vi "Print Console.vi"() -> ()   [LabVIEW 2018]
doc: "인쇄 작업 제출을 컨트롤하고 인쇄 작업의 처리 상태를 모니터"
uses:
  <vilib>/Utility/error.llb/DialogType.ctl
panel:
  out "인쇄 인디케이터":T1={"대기 중"=TRUE, "초기화 중"=FALSE, "인쇄 중"=FALSE, "작업 개수"=""}
  in  "정지 버튼":bool
  in  "큐 이벤트":bool
  out "큐 인쇄 작업":i32(slide) scale=0.0..25.0
  # "큐 인쇄 작업"
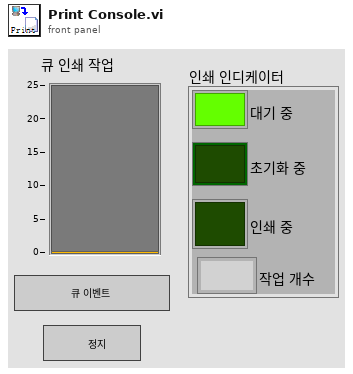
[diagram p1: front panel]
types:
  T1 = cluster{"대기 중":bool, "초기화 중":bool, "인쇄 중":bool, "작업 개수":string}
  T2 = typedef "DialogType.ctl" = u16
  T3 = enum16{"대기", "셋업 초기화", "셋업", "인쇄 초기화", "인쇄", "종료"}
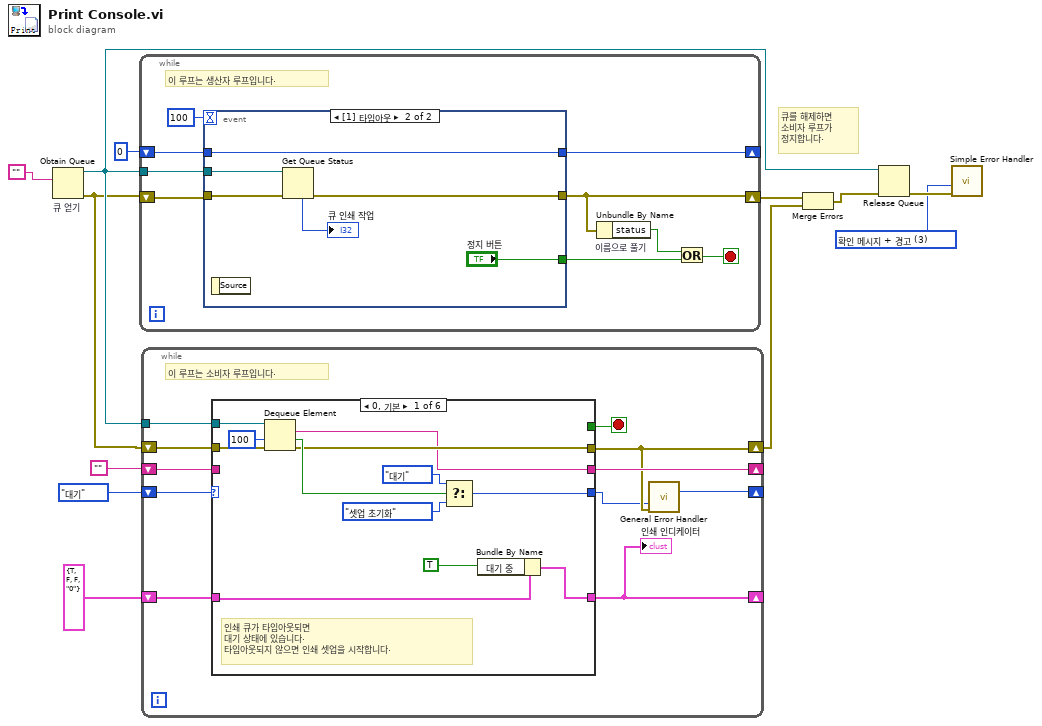
[diagram p0: block diagram]
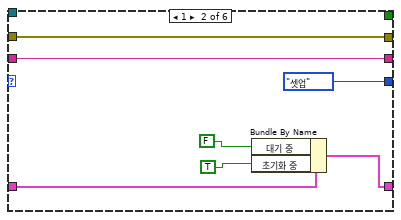
[diagram p2: hidden frame]
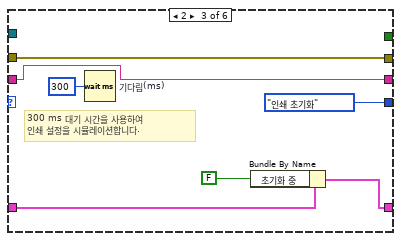
[diagram p3: hidden frame]
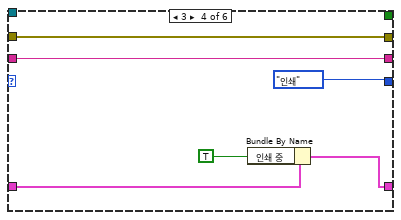
[diagram p4: hidden frame]
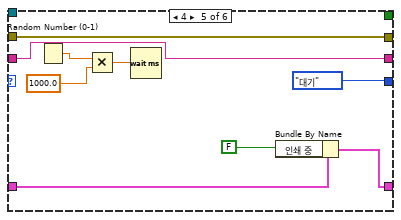
[diagram p5: hidden frame]
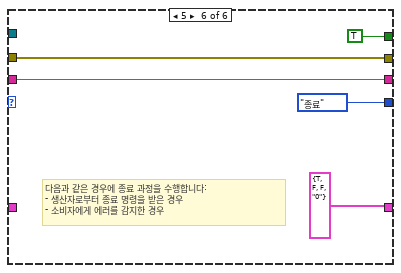
[diagram p6: hidden frame]
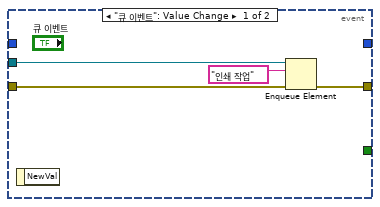
[diagram p7: hidden frame]
diagram:
  w1 = T2 3 items=["대화 상자 없음", "확인 메시지", "메시지 지속 또는 정지", "확인 메시지 + 경고", "지속/정지 + 경고"] ("type of dialog (OK msg:1)")
  # "큐를 해제하면\n소비자 루프가\n정지합니다."
  n1 = Obtain Queue "큐 얻기"(element data type="") -> (queue out=w11:refnum<queue>, error out=w6:errorcluster)  [unwired: 4 in, 1 out]
  n2 = while {
    tunnel: w11 -> [w20]
    shift-right: [w17] -> w5
    shift-left: w6 -> [w19]
    shift-right: [w13] -> _
    shift-left: 0 -> [w14]
    stop <- w18 stop-if-true
    # "이 루프는 생산자 루프입니다."
    n3 = event shown="[1] 타임아웃" {
      selector: _ -> [_ _]
      dyn-events: _ -> [_ _]
      timeout: 100 -> [_ _]
      tunnel: w20 -> [w24 w31]
      tunnel: w19 -> [w23 w30]
      tunnel: [w22 w29] -> w17
      tunnel: [_ "정지 버튼"] -> w15
      tunnel: [_ w27] -> w13
      tunnel: w14 -> [_ w27]
      event "큐 이벤트": Value Change {
        n4 = event-data() -> ()  [unwired: 1 in, 1 out]
        n5 = Enqueue Element(queue=w24, element="인쇄 작업" ("원소"), error in (no error)=w23) -> (error out=w22:errorcluster)  [unwired: 1 in, 2 out]
      }
      event Timeout {
        n6 = event-data() -> ()  [unwired: 1 in, 1 out]
        n7 = Get Queue Status(queue=w31, error in (no error)=w30) -> (error out=w29:errorcluster, # elements in queue=→"큐 인쇄 작업":i32)  [unwired: 1 in, 6 out]
      }
    }
    n8 = Unbundle By Name "이름으로 풀기"(w17) -> ("status"=w16:bool)
    n9 = Or(x=w16, y=w15) -> (x .or. y?=w18:bool)
  }
  n10 = while {
    shift-right: [w39] -> _
    shift-left: T1 {"대기 중"=TRUE, "초기화 중"=FALSE, "인쇄 중"=FALSE, "작업 개수"="0"} ("에러 상수") -> [w40]
    shift-right: [w32] -> _
    shift-left: T3."대기" -> [w42]
    tunnel: w11 -> [w41]
    shift-right: [w37] -> _
    shift-left: "" -> [w36]
    shift-right: [w34] -> w3
    shift-left: w6 -> [w38]
    stop <- w35 stop-if-true
    # "이 루프는 소비자 루프입니다."
    n11 = case shown="0, 기본" w42 {
      tunnel: w41 -> [w53 _ _ _ _ _]
      tunnel: [w52 enum16{"대기", "셋업 초기화", "셋업", "인쇄 초기화", "인쇄"}."셋업" enum16{"대기", "셋업 초기화", "셋업", "인쇄 초기화", "인쇄"}."인쇄 초기화" enum16{"대기", "셋업 초기화", "셋업", "인쇄 초기화", "인쇄"}."인쇄" enum16{"대기", "셋업 초기화", "셋업", "인쇄 초기화", "인쇄"}."대기" T3."종료"] -> w33
      tunnel: [w48 w57 w65 w72 w79 T1 {"대기 중"=TRUE, "초기화 중"=FALSE, "인쇄 중"=FALSE, "작업 개수"="0"} ("에러 상수")] -> w39
      tunnel: w40 -> [w47 w60 w66 w73 w80 _]
      tunnel: w38 -> [w45 w56 w63 w70 w76 w86]
      tunnel: [w44 w56 w63 w70 w76 w86] -> w34
      tunnel: [w43 w55 w62 w69 w75 w87] -> w37
      tunnel: w36 -> [_ w55 w62 w69 w75 w87]
      tunnel: [_ _ _ _ _ TRUE] -> w35
      frame 0, Default {
        # "인쇄 큐가 타임아웃되면\n대기 상태에 있습니다.\n타임아웃되지 않으면 인쇄 셋업을 시작합니다."
        n12 = Dequeue Element(queue=w53, timeout in ms (-1)=100 ("타임아웃(ms) (-1)"), error in (no error)=w45) -> (element=w43:string, timed out?=w51:bool, error out=w44:errorcluster)  [unwired: 1 out]
        n13 = Select(t=enum16{"대기", "셋업 초기화", "셋업", "인쇄 초기화", "인쇄"}."대기", s=w51, f=enum16{"대기", "셋업 초기화", "셋업", "인쇄 초기화", "인쇄"}."셋업 초기화") -> (s? t:f=w52:enum16{"대기", "셋업 초기화", "셋업", "인쇄 초기화", "인쇄"})
        n14 = Bundle By Name(cluster=w47, "대기 중"=TRUE) -> (w48:T1)
      }
      frame 1 {
        n15 = Bundle By Name(cluster=w60, "대기 중"=FALSE, "초기화 중"=TRUE) -> (w57:T1)
      }
      frame 2 {
        # "300 ms 대기 시간을 사용하여\n인쇄 설정을 시뮬레이션합니다."
        n16 = Wait (ms) "기다림(ms)"(milliseconds to wait=u32 300 ("대기 시간 (ms)")) -> ()  [unwired: 1 out]
        n17 = Bundle By Name(cluster=w66, "초기화 중"=FALSE) -> (w65:T1)
      }
      frame 3 {
        n18 = Bundle By Name(cluster=w73, "인쇄 중"=TRUE) -> (w72:T1)
      }
      frame 4 {
        n19 = Random Number (0-1)() -> (number: 0 to 1=w83:dbl)
        n20 = Multiply(x=w83, y=1000.0) -> (x*y=w81:dbl)
        n21 = Wait (ms)(milliseconds to wait=w81) -> ()  [unwired: 1 out]
        n22 = Bundle By Name(cluster=w80, "인쇄 중"=FALSE) -> (w79:T1)
      }
      frame 5 {
        # "다음과 같은 경우에 종료 과정을 수행합니다:\n- 생산자로부터 종료 명령을 받은 경우\n- 소비자에게 에러를 감지한 경우"
      }
    }
    "인쇄 인디케이터" <- w39
    n23 = call <vilib>:"General Error Handler.vi"("type of dialog (OK msg:1)"=w33, "error in (no error)"=w34) -> ("code out"=w32:i32)  [unwired: 9 in, 4 out]
  }
  n24 = Merge Errors(w5, w3) -> (w4:errorcluster)
  n25 = Release Queue(queue=w11, error in (no error)=w4) -> (error out=w2:errorcluster)  [unwired: 1 in, 2 out]
  n26 = call <vilib>:"Simple Error Handler.vi"("type of dialog (OK msg:1)"=w1, "error in (no error)"=w2) -> ()  [unwired: 3 in, 5 out]
